vi "Change Language.vi"(9 "Array IN":string[][](array[string]), 10 "References Pane":T1(array[cluster]), 11 "Langues/Languages":u8) -> ()   [LabVIEW 2013, in "main.lvlib"]
doc: "Jean-Marc Simard \nExaprom inc. 2009"
uses:
  main.lvlib
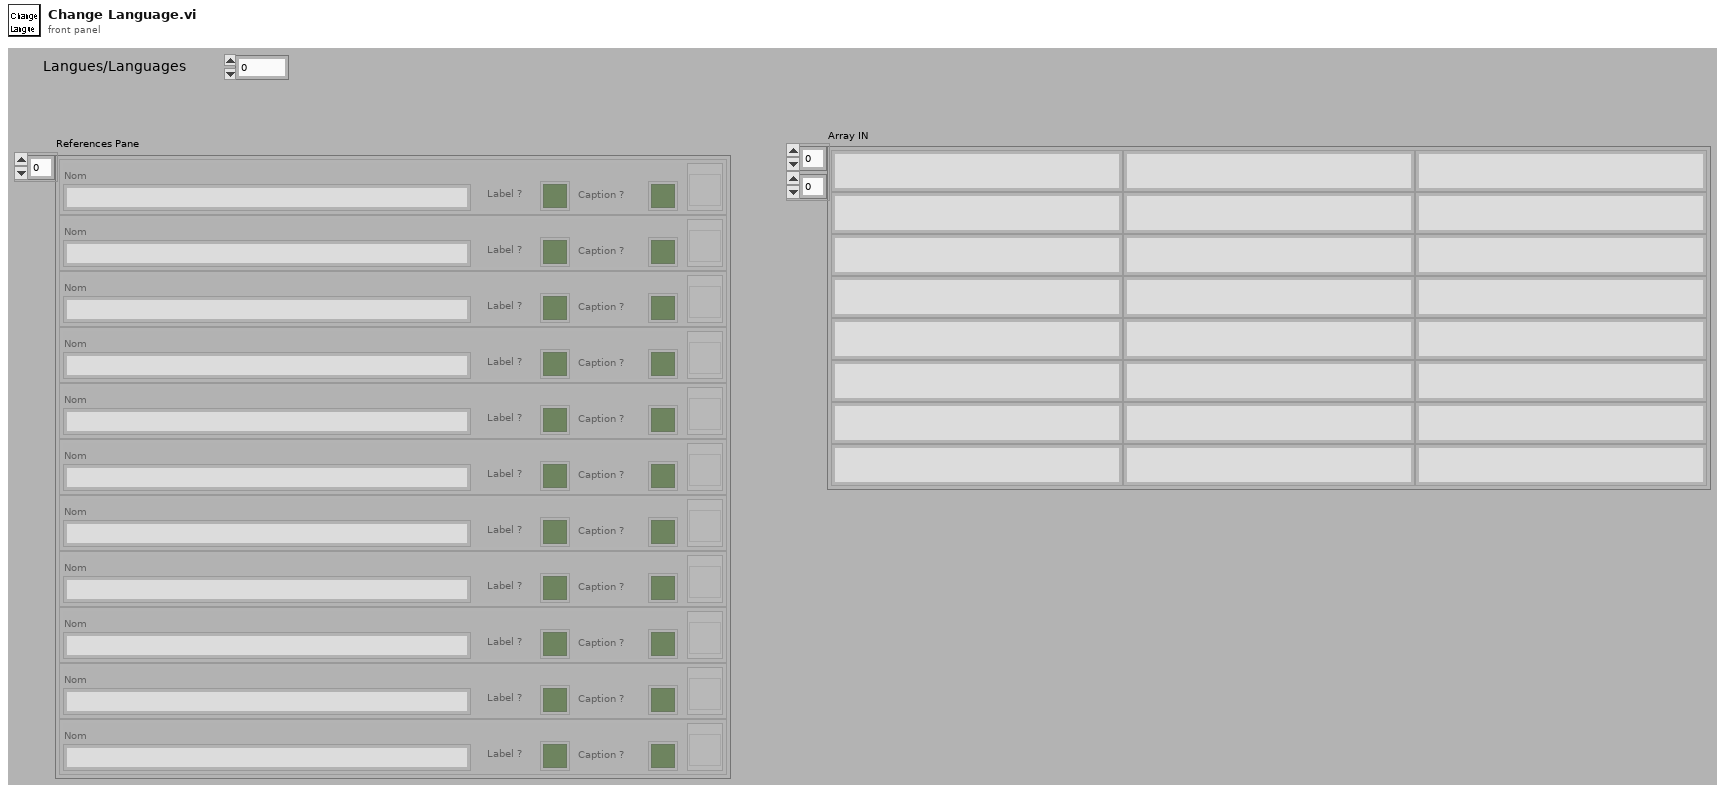
[diagram p1: front panel]
types:
  T1 = cluster{"Nom":string, "Label ?":bool, "Caption ?":bool, "Ref":refnum<vi>}[]
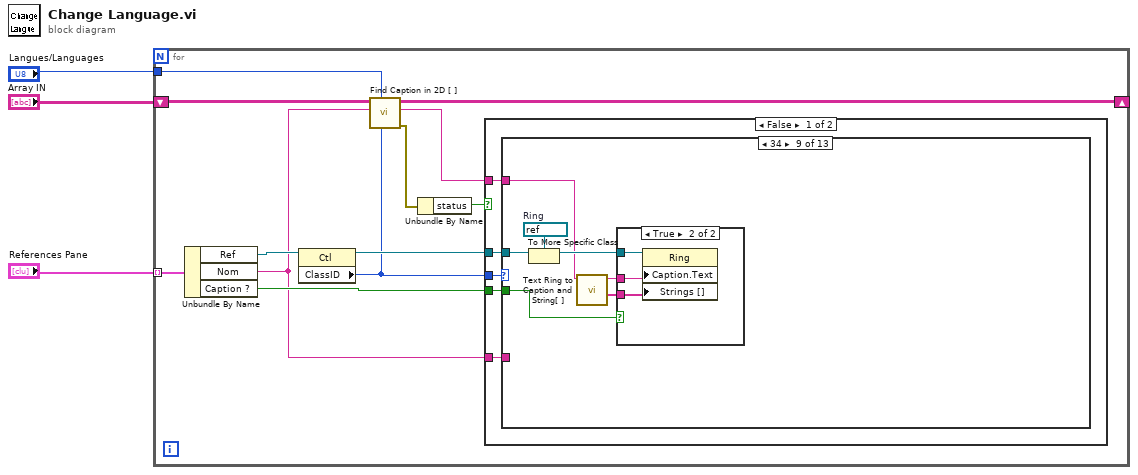
[diagram p0: block diagram]
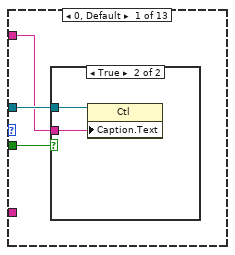
[diagram p2: hidden frame]
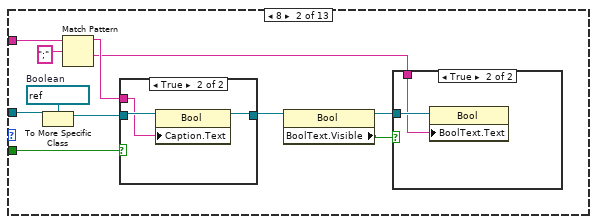
[diagram p4: hidden frame]
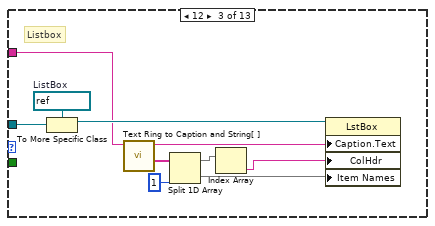
[diagram p7: hidden frame]
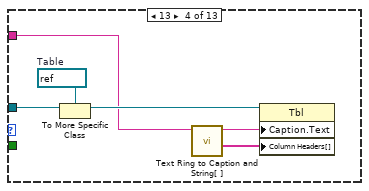
[diagram p8: hidden frame]
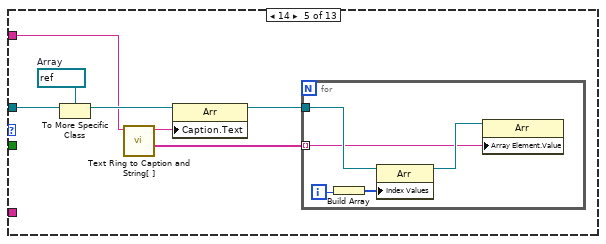
[diagram p9: hidden frame]
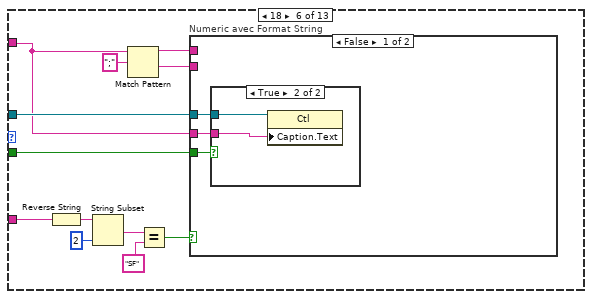
[diagram p10: hidden frame]
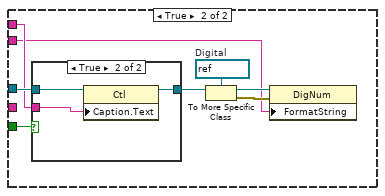
[diagram p12: hidden frame]
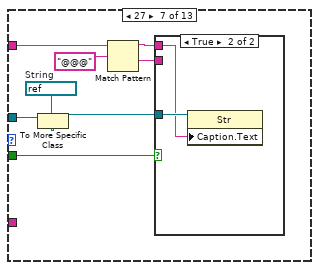
[diagram p14: hidden frame]
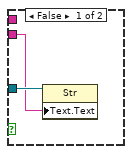
[diagram p15: hidden frame]
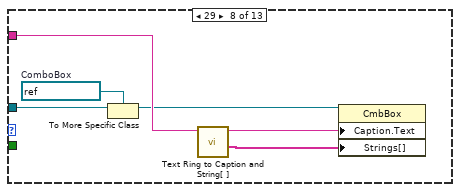
[diagram p16: hidden frame]
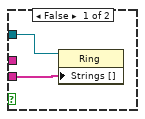
[diagram p17: hidden frame]
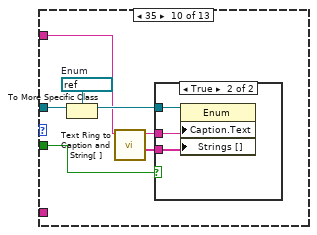
[diagram p18: hidden frame]
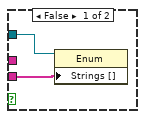
[diagram p19: hidden frame]
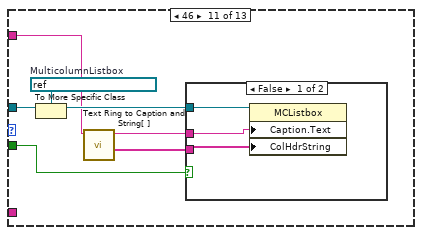
[diagram p20: hidden frame]
diagram:
  n1 = for {
    tunnel: "References Pane" -> [w5] mode=indexing
    shift-right: [w13] -> _
    shift-left: "Array IN" -> [w14]
    tunnel: "Langues/Languages" -> [w6]
    n2 = Unbundle By Name(w5) -> ("Ref"=w15:refnum<vi>, "Nom"=w4:string, "Caption ?"=w9:bool)
    n3 = property class="Ctl"(reference=w15) -> (reference out=w10:refnum<vi>, "ClassID"=w8:u32)  [unwired: 1 in, 1 out]
    n4 = call "Find Caption in 2D [ ].vi"("Class ID"=w8, "Langues/Languages"=w6, "Nom"=w4, "Array IN"=w14) -> ("error out"=w12:errorcluster, "Légende"=w11:string, "Array OUT"=w13:string[][])  [unwired: 5 in]
    n5 = Unbundle By Name(w12) -> ("status"=w7:bool)
    n6 = case shown="False" w7 {
      tunnel: w10 -> [w20 _]
      tunnel: w11 -> [w19 _]
      tunnel: w8 -> [w18 _]
      tunnel: w9 -> [w17 _]
      tunnel: w4 -> [w16 _]
      frame False {
        n7 = case shown="34" w18 {
          tunnel: w20 -> [w23 w36 w51 w57 w64 w77 w106 w116 w123 w135 w147 w157 w161]
          tunnel: w19 -> [w22 w33 w49 w55 w62 w74 w103 w115 w120 w132 w144 w158 w162]
          tunnel: w17 -> [w21 w32 _ _ _ w76 w104 _ w121 w133 w145 _ _]
          tunnel: w16 -> [_ _ _ _ _ w71 _ _ _ _ _ _ _]
          frame 0, Default {
            n8 = case shown="True" w21 {
              tunnel: w23 -> [_ w25]
              tunnel: w22 -> [_ w24]
              frame False {
              }
              frame True {
                n9 = property class="Ctl"(reference=w25, "Caption.Text"=w24) -> ()  [unwired: 1 in, 2 out]
              }
            }
          }
          frame 8 {
            w35 = refnum<vi> refnum  # Boolean
            n10 = To More Specific Class(target class=w35, reference=w36) -> (specific class reference=w30:refnum<vi>)  [unwired: 1 in, 1 out]
            n11 = Match Pattern(string=w33, regular expression=";") -> (before substring=w31:string, after substring=w26:string)  [unwired: 3 out]
            n12 = case shown="True" w32 {
              tunnel: w31 -> [_ w41]
              tunnel: w30 -> [w39 w42]
              tunnel: [w39 w40] -> w29
              frame False {
              }
              frame True {
                n13 = property class="Bool"(reference=w42, "Caption.Text"=w41) -> (reference out=w40:refnum<vi>)  [unwired: 1 in, 1 out]
              }
            }
            n14 = property class="Bool"(reference=w29) -> (reference out=w27:refnum<vi>, "BoolText.Visible"=w28:bool)  [unwired: 1 in, 1 out]
            n15 = case shown="True" w28 {
              tunnel: w27 -> [_ w38]
              tunnel: w26 -> [_ w37]
              frame False {
              }
              frame True {
                n16 = property class="Bool"(reference=w38, "BoolText.Text"=w37) -> ()  [unwired: 1 in, 2 out]
              }
            }
          }
          frame 12 {
            w52 = refnum<vi> refnum  # ListBox
            # "Listbox"
            n17 = To More Specific Class(target class=w52, reference=w51) -> (specific class reference=w50:refnum<vi>)  [unwired: 1 in, 1 out]
            n18 = call "Text Ring to Caption and String[ ].vi"("String"=w49) -> ("String[ ]"=w47:string[], "Caption"=w48:string)  [unwired: 1 in, 8 out]
            n19 = Split 1D Array(array=w47, index=1) -> (first subarray=w44:string[], second subarray=w45:string[])
            n20 = Index Array(array=w44) -> (element=w43:string)  [unwired: 1 in]
            n21 = property class="LstBox"(reference=w50, "Caption.Text"=w48, "ColHdr"=w43, "Item Names"=w45) -> ()  [unwired: 1 in, 2 out]
          }
          frame 13 {
            w58 = refnum<vi> refnum  # Table
            n22 = To More Specific Class(target class=w58, reference=w57) -> (specific class reference=w56:refnum<vi>)  [unwired: 1 in, 1 out]
            n23 = call "Text Ring to Caption and String[ ].vi"("String"=w55) -> ("String[ ]"=w53:string[], "Caption"=w54:string)  [unwired: 1 in, 8 out]
            n24 = property class="Tbl"(reference=w56, "Caption.Text"=w54, "Column Headers[]"=w53) -> ()  [unwired: 1 in, 2 out]
          }
          frame 14 {
            w65 = refnum<vi> refnum  # Array
            n25 = To More Specific Class(target class=w65, reference=w64) -> (specific class reference=w63:refnum<vi>)  [unwired: 1 in, 1 out]
            n26 = call "Text Ring to Caption and String[ ].vi"("String"=w62) -> ("String[ ]"=w59:string[], "Caption"=w61:string)  [unwired: 1 in, 8 out]
            n27 = property class="Arr"(reference=w63, "Caption.Text"=w61) -> (reference out=w60:refnum<vi>)  [unwired: 1 in, 1 out]
            n28 = for {
              tunnel: w60 -> [w70]
              tunnel: w59 -> [w66] mode=indexing
              i -> [w68]
              n29 = Build Array(w68) -> (w69:i32[])
              n30 = property class="Arr"(reference=w70, "Index Values"=w69) -> (reference out=w67:refnum<vi>)  [unwired: 1 in, 1 out]
              n31 = property class="Arr"(reference=w67, "Array Element.Value"=w66) -> ()  [unwired: 1 in, 2 out]
            }
          }
          frame 18 {
            n32 = Reverse String(1:w71) -> (0:w82:string)
            n33 = String Subset(string=w82, length (rest)=2 ("length (rest)")) -> (substring=w80:string)  [unwired: 1 out]
            n34 = Match Pattern(string=w74, regular expression=";") -> (before substring=w73:string, after substring=w72:string)  [unwired: 3 out]
            n35 = Equal?(x=w80, y="SF") -> (x = y?=w78:bool)
            n36 = case "Numeric avec Format String" shown="False" w78 {
              tunnel: w77 -> [w85 w95]
              tunnel: w74 -> [w84 _]
              tunnel: w76 -> [w83 w94]
              tunnel: w73 -> [_ w93]
              tunnel: w72 -> [_ w88]
              frame False {
                n37 = case shown="True" w83 {
                  tunnel: w85 -> [_ w87]
                  tunnel: w84 -> [_ w86]
                  frame False {
                  }
                  frame True {
                    n38 = property class="Ctl"(reference=w87, "Caption.Text"=w86) -> ()  [unwired: 1 in, 2 out]
                  }
                }
              }
              frame True {
                w89 = refnum<vi> refnum  # Digital
                n39 = case shown="True" w94 {
                  tunnel: w95 -> [w96 w99]
                  tunnel: w93 -> [_ w98]
                  tunnel: [w96 w97] -> w90
                  frame False {
                  }
                  frame True {
                    n40 = property class="Ctl"(reference=w99, "Caption.Text"=w98) -> (reference out=w97:refnum<vi>)  [unwired: 1 in, 1 out]
                  }
                }
                n41 = To More Specific Class(target class=w89, reference=w90) -> (specific class reference=w91:refnum<vi>, error out=w92:errorcluster)  [unwired: 1 in]
                n42 = property class="DigNum"(reference=w91, error in=w92, "FormatString"=w88) -> ()  [unwired: 2 out]
              }
            }
          }
          frame 27 {
            w107 = refnum<vi> refnum  # String
            n43 = To More Specific Class(target class=w107, reference=w106) -> (specific class reference=w105:refnum<vi>)  [unwired: 1 in, 1 out]
            n44 = Match Pattern(string=w103, regular expression="@@@") -> (before substring=w100:string, after substring=w101:string)  [unwired: 3 out]
            n45 = case shown="True" w104 {
              tunnel: w105 -> [w109 w111]
              tunnel: w101 -> [w108 _]
              tunnel: w100 -> [_ w110]
              frame False {
                n46 = property class="Str"(reference=w109, "Text.Text"=w108) -> ()  [unwired: 1 in, 2 out]
              }
              frame True {
                n47 = property class="Str"(reference=w111, "Caption.Text"=w110) -> ()  [unwired: 1 in, 2 out]
              }
            }
          }
          frame 29 {
            w117 = refnum<vi> refnum  # ComboBox
            n48 = To More Specific Class(target class=w117, reference=w116) -> (specific class reference=w114:refnum<vi>)  [unwired: 1 in, 1 out]
            n49 = call "Text Ring to Caption and String[ ].vi"("String"=w115) -> ("String[ ]"=w112:string[], "Caption"=w113:string)  [unwired: 1 in, 8 out]
            n50 = property class="CmbBox"(reference=w114, "Caption.Text"=w113, "Strings[]"=w112) -> ()  [unwired: 1 in, 2 out]
          }
          frame 34 {
            w124 = refnum<vi> refnum  # Ring
            n51 = To More Specific Class(target class=w124, reference=w123) -> (specific class reference=w122:refnum<vi>)  [unwired: 1 in, 1 out]
            n52 = call "Text Ring to Caption and String[ ].vi"("String"=w120) -> ("String[ ]"=w119:string[], "Caption"=w118:string)  [unwired: 1 in, 8 out]
            n53 = case shown="True" w121 {
              tunnel: w122 -> [w126 w129]
              tunnel: w119 -> [w125 w127]
              tunnel: w118 -> [_ w128]
              frame False {
                n54 = property class="Ring"(reference=w126, "Strings []"=w125) -> ()  [unwired: 1 in, 2 out]
              }
              frame True {
                n55 = property class="Ring"(reference=w129, "Caption.Text"=w128, "Strings []"=w127) -> ()  [unwired: 1 in, 2 out]
              }
            }
          }
          frame 35 {
            w136 = refnum<vi> refnum  # Enum
            n56 = To More Specific Class(target class=w136, reference=w135) -> (specific class reference=w134:refnum<vi>)  [unwired: 1 in, 1 out]
            n57 = call "Text Ring to Caption and String[ ].vi"("String"=w132) -> ("String[ ]"=w131:string[], "Caption"=w130:string)  [unwired: 1 in, 8 out]
            n58 = case shown="True" w133 {
              tunnel: w134 -> [w138 w141]
              tunnel: w131 -> [w137 w139]
              tunnel: w130 -> [_ w140]
              frame False {
                n59 = property class="Enum"(reference=w138, "Strings []"=w137) -> ()  [unwired: 1 in, 2 out]
              }
              frame True {
                n60 = property class="Enum"(reference=w141, "Caption.Text"=w140, "Strings []"=w139) -> ()  [unwired: 1 in, 2 out]
              }
            }
          }
          frame 46 {
            w148 = refnum<vi> refnum  # MulticolumnListbox
            n61 = To More Specific Class(target class=w148, reference=w147) -> (specific class reference=w146:refnum<vi>)  [unwired: 1 in, 1 out]
            n62 = call "Text Ring to Caption and String[ ].vi"("String"=w144) -> ("String[ ]"=w143:string[], "Caption"=w142:string)  [unwired: 1 in, 8 out]
            n63 = case shown="False" w145 {
              tunnel: w146 -> [w151 w154]
              tunnel: w143 -> [w149 w152]
              tunnel: w142 -> [w150 w153]
              frame False {
                n64 = property class="MCListbox"(reference=w151, "Caption.Text"=w150, "ColHdrString"=w149) -> ()  [unwired: 1 in, 2 out]
              }
              frame True {
                n65 = property class="MCListbox"(reference=w154, "Caption.Text"=w153, "ColHdrString"=w152) -> ()  [unwired: 1 in, 2 out]
              }
            }
          }
          frame 55 {
            w155 = refnum<vi> refnum  # TabControl
            n66 = To More Specific Class(target class=w155, reference=w157) -> (specific class reference=w156:refnum<vi>)  [unwired: 1 in, 1 out]
            n67 = call "Name Tab Control.vi"("TabCtl Refnum"=w156, "String"=w158) -> ()  [unwired: 10 in]
          }
          frame 83 {
            n68 = To More Specific Class(target class=refnum<vi> refnum ("XYGraph Refnum"), reference=w161) -> (specific class reference=w160:refnum<vi>)  [unwired: 1 in, 1 out]
            n69 = call "Axes XY Graph.vi"("XYGraph Refnum"=w160, "String"=w162) -> ()  [unwired: 10 out]
          }
        }
      }
      frame True {
      }
    }
  }
